vi "AccumulateDataNoPWM.vi"(0 "Current In":dbl[](array[numeric]), 1 "Thrust In":dbl[](array[numeric]), 2 "RPM In":dbl[](array[numeric]), 3 "Power In":dbl[](array[numeric]), 4 "Temperature In":dbl[](array[numeric]), 5 "Voltage In":dbl[](array[numeric]), 6 "Noise In":dbl[](array[numeric]), 7 "Data":T1) -> (20 "Current Out":dbl[](array[numeric]), 21 "Thrust Out":dbl[](array[numeric]), 22 "RPM Out":dbl[](array[numeric]), 23 "Power Out":dbl[](array[numeric]), 24 "Temperature Out":dbl[](array[numeric]), 25 "Voltage Out":dbl[](array[numeric]), 26 "Noise Out":dbl[](array[numeric]))   [LabVIEW 2023]
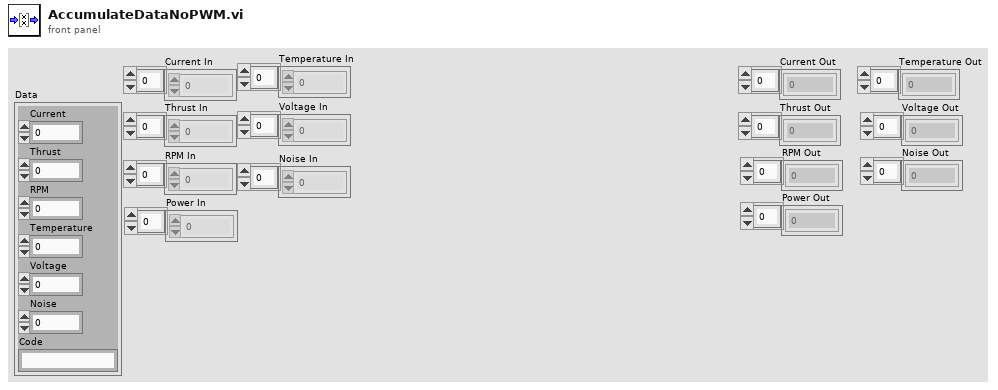
[diagram p1: front panel]
types:
  T1 = cluster{"Current":dbl, "Thrust":dbl, "RPM":dbl, "Temperature":dbl, "Voltage":dbl, "Noise":dbl, "Code":string}
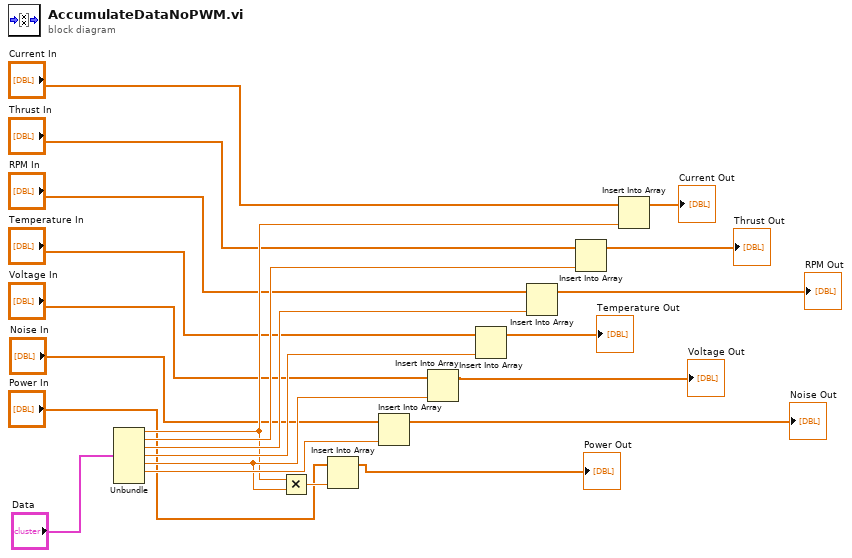
[diagram p0: block diagram]
diagram:
  n1 = Unbundle("Data") -> ("Current"=w17:dbl, "Thrust"=w18:dbl, "RPM"=w19:dbl, "Temperature"=w20:dbl, "Voltage"=w21:dbl, "Noise"=w22:dbl)  [unwired: 1 out]
  n2 = Multiply(x=w17, y=w21) -> (x*y=w16:dbl)
  n3 = Insert Into Array(array="Power In", new element=w16) -> (→"Power Out":dbl[])  [unwired: 1 in]
  n4 = Insert Into Array(array="Noise In", new element=w22) -> (→"Noise Out":dbl[])  [unwired: 1 in]
  n5 = Insert Into Array(array="Voltage In", new element=w21) -> (→"Voltage Out":dbl[])  [unwired: 1 in]
  n6 = Insert Into Array(array="Temperature In", new element=w20) -> (→"Temperature Out":dbl[])  [unwired: 1 in]
  n7 = Insert Into Array(array="RPM In", new element=w19) -> (→"RPM Out":dbl[])  [unwired: 1 in]
  n8 = Insert Into Array(array="Thrust In", new element=w18) -> (→"Thrust Out":dbl[])  [unwired: 1 in]
  n9 = Insert Into Array(array="Current In", new element=w17) -> (→"Current Out":dbl[])  [unwired: 1 in]
